vi "Day 06 Part 1.vi"(11 "Input":string) -> (3 "Output":dbl)   [LabVIEW 2021]
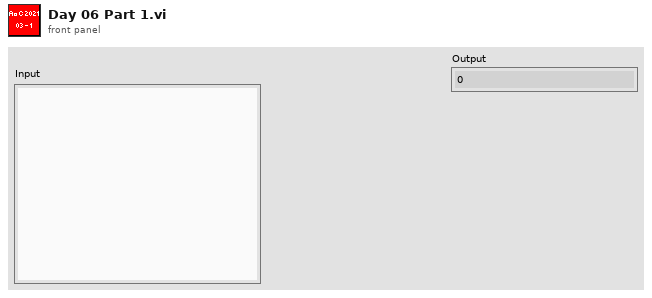
[diagram p1: front panel]
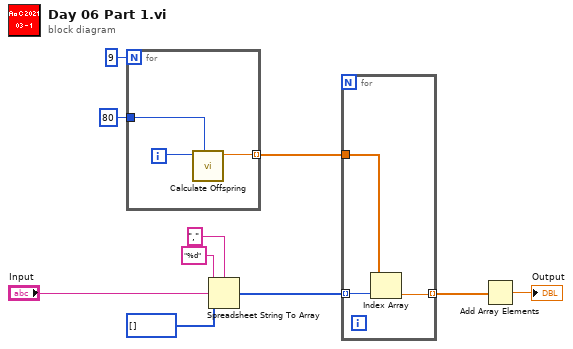
[diagram p0: block diagram]
diagram:
  n1 = for {
    N: 9 -> [_]
    tunnel: 80 -> [w12]
    tunnel: [w11] -> w3 mode=indexing
    i -> [w13]
    n2 = call "Calculate Offspring.vi"("Days"=w12, "Age"=w13) -> ("Offspring"=w11:dbl)  [unwired: 9 in]
  }
  n3 = Spreadsheet String To Array(delimiter (Tab)=",", format string="%d", spreadsheet string="Input", array type (2D Dbl)=i32[] []) -> (array=w4:i32[])
  n4 = for {
    tunnel: w4 -> [w16] mode=indexing
    tunnel: w3 -> [w15]
    tunnel: [w14] -> w1 mode=indexing
    n5 = Index Array(array=w15, index=w16) -> (element=w14:dbl)
  }
  n6 = Add Array Elements(numeric array=w1) -> (sum=→"Output":dbl)
